vi "DSF.Engine.Memory.ObjectPool.Set Object.vi"(8 "error in (no error)":errorcluster, 9 "Object":refnum<class>, 10 "index":i32, 11 "ObjectPool in":refnum<class "DSF.Engine.Memory.ObjectPool.lvclass">) -> (0 "error out":errorcluster, 3 "ObjectPool out":refnum<class "DSF.Engine.Memory.ObjectPool.lvclass">)   [LabVIEW 2016, in "DSF.Engine.lvlib" / "DSF.Engine.Memory.ObjectPool.lvclass"]
uses:
  DSF.Engine.Memory.ObjectPool.lvclass
  DSF.Engine.Memory.ObjectPool.lvclass/DSF.Engine.Memory.ObjectPool.ctl
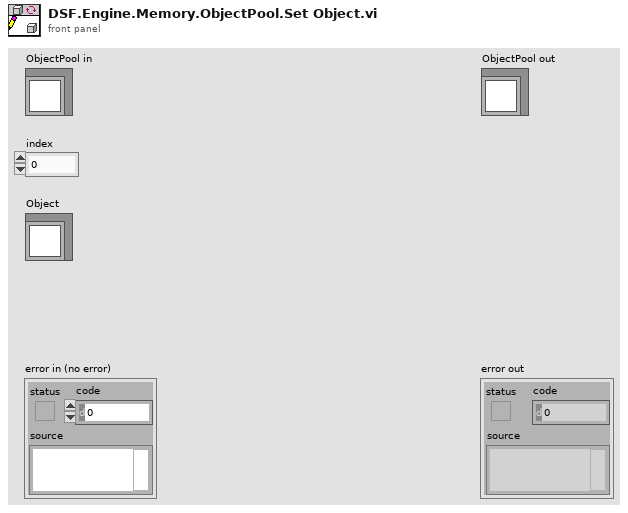
[diagram p1: front panel]
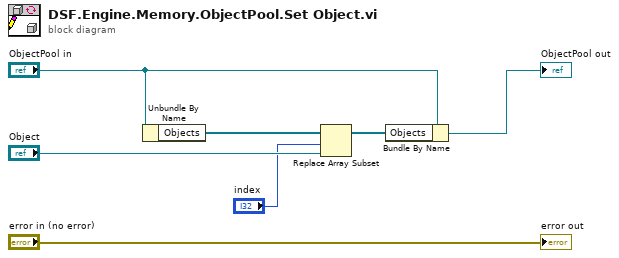
[diagram p0: block diagram]
diagram:
  n1 = Unbundle By Name("ObjectPool in") -> ("Objects"=w3:refnum<class>[])
  n2 = Replace Array Subset(array=w3, new element="Object", index="index") -> (w2:refnum<class>[])
  n3 = Bundle By Name(cluster="ObjectPool in", "Objects"=w2) -> (→"ObjectPool out":refnum<class "DSF.Engine.Memory.ObjectPool.lvclass">)
  "error out" <- "error in (no error)"
